vi "whoWins.vi"(2 "white":bool[][](array[boolean]), 3 "black":bool[][](array[boolean])) -> (0 "wWins":bool, 1 "bWins":bool)   [LabVIEW 2014]
panel:
  in  "/wWins":bool
  in  "/bWins":bool
  in  "\\wWins":bool
  in  "\\bWins":bool
  in  "|wWins":bool
  in  "|bWins":bool
  in  "-wWins":bool
  in  "-bWins":bool
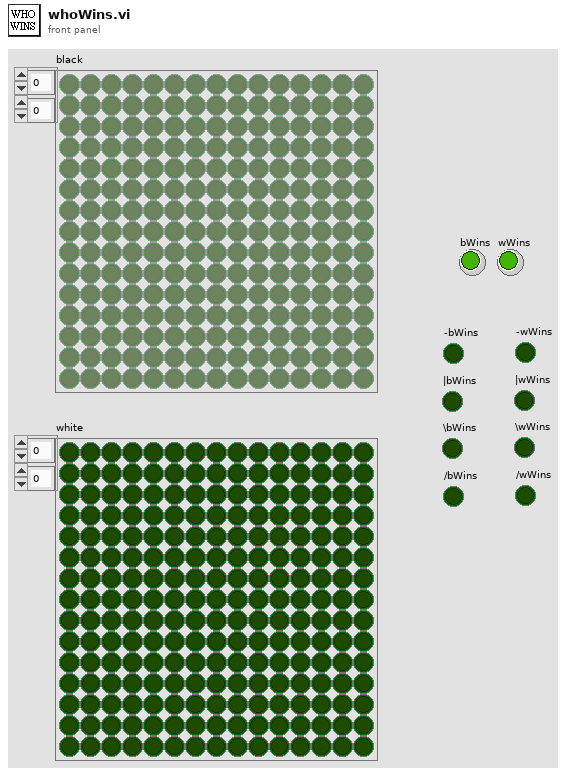
[diagram p1: front panel]
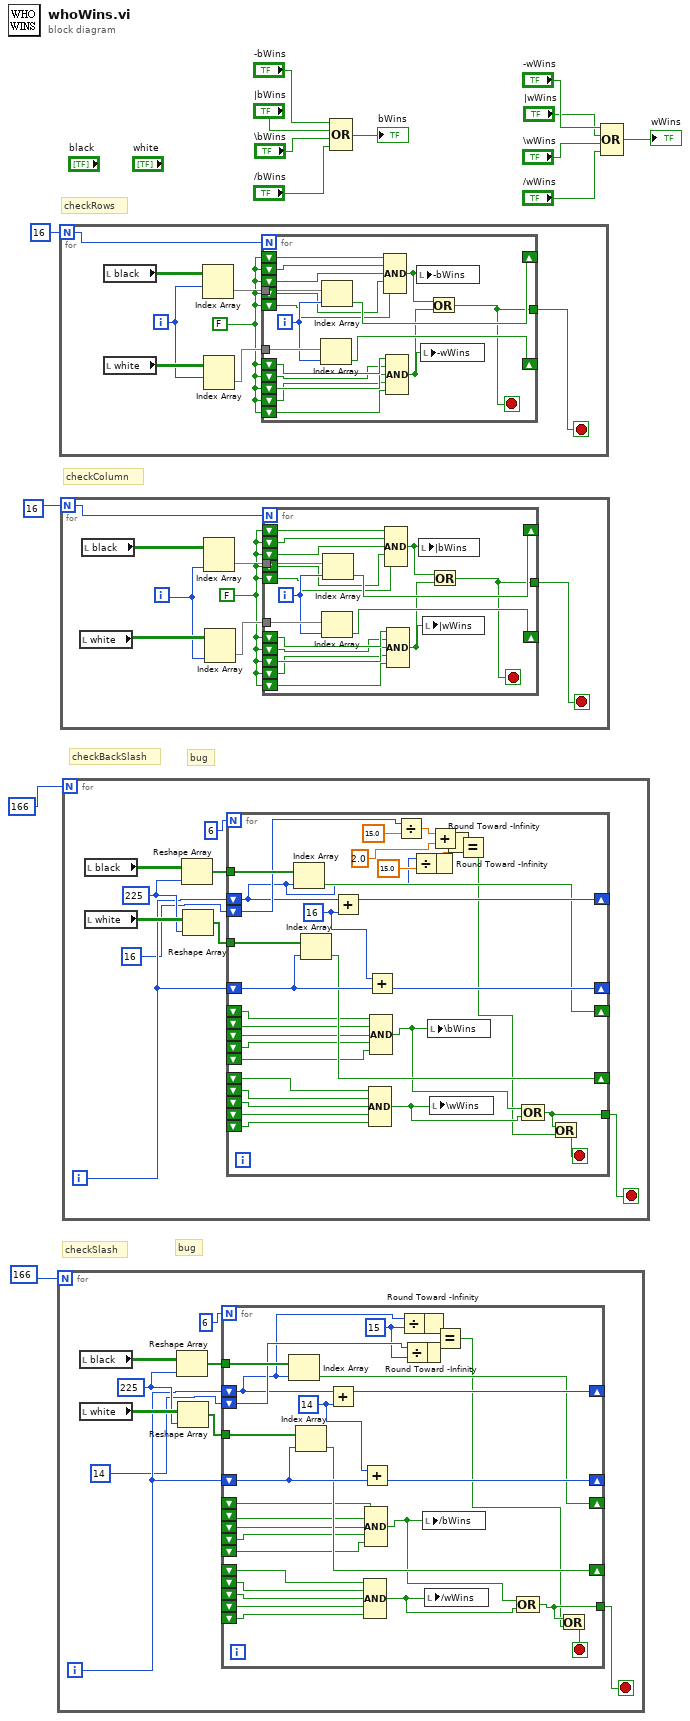
[diagram p0: block diagram]
diagram:
  # "bug"
  # "bug"
  # "checkSlash"
  # "checkBackSlash"
  # "checkColumn"
  # "checkRows"
  n1 = for {
    N: 166 -> [_]
    i -> [w16]
    stop <- w18 stop-if-true
    w21 = 225
    n2 = local read "black"() -> (w23:bool[][])
    n3 = local read "white"() -> (w22:bool[][])
    n4 = Reshape Array(w23, w21) -> (w17:bool[])
    n5 = Reshape Array(w22, w21) -> (w20:bool[])
    n6 = for {
      N: 6 -> [_]
      tunnel: w17 -> [w53]
      tunnel: w20 -> [w52]
      shift-right: [w51] -> _
      shift-left: w16 -> [w29]
      shift-right: [w50] -> _
      shift-left: w16 -> [w48]
      shift-right: [w47] -> _
      shift-left: _ -> [w45]
      shift-right: [w46] -> _
      shift-left: _ -> [w40]
      shift-left: _ -> [w44]
      shift-left: _ -> [w43]
      shift-left: _ -> [w42]
      shift-left: _ -> [w41]
      shift-left: _ -> [w39]
      shift-left: _ -> [w38]
      shift-left: _ -> [w37]
      shift-left: _ -> [w36]
      tunnel: [w33] -> w18
      shift-left: 14 -> [w30]
      stop <- w28 stop-if-true
      w26 = 15
      w49 = 14
      n7 = Index Array(array=w53, index=w29) -> (element=w47:bool)
      n8 = Index Array(array=w52, index=w48) -> (element=w46:bool)
      n9 = Add(x=w29, y=w49) -> (x+y=w51:i32)
      n10 = Add(x=w49, y=w48) -> (x+y=w50:i32)
      n11 = Compound Arithmetic op=AND(w40, w39, w38, w37, w36) -> (w34:bool)
      n12 = Compound Arithmetic op=AND(w45, w44, w43, w42, w41) -> (w35:bool)
      n13 = Divide(x=w29, y=w26) -> (x/y=w32:dbl)
      n14 = Divide(x=w30, y=w26) -> (x/y=w31:dbl)
      n15 = Round Toward -Infinity(1:w31) -> (0:w24:dbl)
      n16 = Round Toward -Infinity(1:w32) -> (0:w25:dbl)
      n17 = local write "/bWins"(w35) -> ()
      n18 = local write "/wWins"(w34) -> ()
      n19 = Equal?(x=w25, y=w24) -> (x = y?=w27:bool)
      n20 = Compound Arithmetic op=OR(w35, w34) -> (w33:bool)
      n21 = Or(x=w33, y=w27) -> (x .or. y?=w28:bool)
    }
  }
  n22 = for {
    N: 16 -> [w55]
    i -> [w59]
    stop <- w56 stop-if-true
    w54 = FALSE
    n23 = local read "black"() -> (w61:bool[][])
    n24 = local read "white"() -> (w60:bool[][])
    n25 = Index Array(array=w61, index (row)=w59) -> (element=w58:bool[])  [unwired: 1 in]
    n26 = Index Array(array=w60, index (row)=w59) -> (element=w57:bool[])  [unwired: 1 in]
    n27 = for {
      N: w55 -> [_]
      tunnel: w58 -> [w78]
      tunnel: w57 -> [w79]
      shift-right: [w76] -> _
      shift-left: w54 -> [w74]
      shift-right: [w75] -> _
      shift-left: w54 -> [w69]
      shift-left: w54 -> [w68]
      shift-left: w54 -> [w67]
      shift-left: w54 -> [w66]
      shift-left: w54 -> [w65]
      shift-left: w54 -> [w73]
      shift-left: w54 -> [w72]
      shift-left: w54 -> [w71]
      shift-left: w54 -> [w70]
      tunnel: [w62] -> w56
      i -> [w77]
      stop <- w62 stop-if-true
      n28 = Index Array(array=w79, index=w77) -> (element=w75:bool)
      n29 = Index Array(array=w78, index=w77) -> (element=w76:bool)
      n30 = Compound Arithmetic op=AND(w74, w73, w72, w71, w70) -> (w64:bool)
      n31 = Compound Arithmetic op=AND(w69, w68, w67, w66, w65) -> (w63:bool)
      n32 = local write "-bWins"(w64) -> ()
      n33 = local write "-wWins"(w63) -> ()
      n34 = Or(x=w64, y=w63) -> (x .or. y?=w62:bool)
    }
  }
  n35 = for {
    N: 16 -> [w81]
    i -> [w82]
    stop <- w85 stop-if-true
    w80 = FALSE
    n36 = local read "white"() -> (w84:bool[][])
    n37 = local read "black"() -> (w83:bool[][])
    n38 = Index Array(array=w83, index (col)=w82) -> (element=w87:bool[])  [unwired: 1 in]
    n39 = Index Array(array=w84, index (col)=w82) -> (element=w86:bool[])  [unwired: 1 in]
    n40 = for {
      N: w81 -> [_]
      tunnel: w87 -> [w104]
      tunnel: w86 -> [w105]
      shift-right: [w102] -> _
      shift-left: w80 -> [w100]
      shift-right: [w101] -> _
      shift-left: w80 -> [w95]
      shift-left: w80 -> [w94]
      shift-left: w80 -> [w93]
      shift-left: w80 -> [w92]
      shift-left: w80 -> [w91]
      shift-left: w80 -> [w99]
      shift-left: w80 -> [w98]
      shift-left: w80 -> [w97]
      shift-left: w80 -> [w96]
      tunnel: [w88] -> w85
      i -> [w103]
      stop <- w88 stop-if-true
      n41 = Index Array(array=w105, index=w103) -> (element=w101:bool)
      n42 = Index Array(array=w104, index=w103) -> (element=w102:bool)
      n43 = Compound Arithmetic op=AND(w100, w99, w98, w97, w96) -> (w90:bool)
      n44 = Compound Arithmetic op=AND(w95, w94, w93, w92, w91) -> (w89:bool)
      n45 = local write "|bWins"(w90) -> ()
      n46 = local write "|wWins"(w89) -> ()
      n47 = Or(x=w90, y=w89) -> (x .or. y?=w88:bool)
    }
  }
  n48 = for {
    N: 166 -> [_]
    i -> [w107]
    stop <- w109 stop-if-true
    w112 = 225
    n49 = local read "black"() -> (w114:bool[][])
    n50 = local read "white"() -> (w113:bool[][])
    n51 = Reshape Array(w114, w112) -> (w108:bool[])
    n52 = Reshape Array(w113, w112) -> (w111:bool[])
    n53 = for {
      N: 6 -> [_]
      tunnel: w108 -> [w147]
      tunnel: w111 -> [w146]
      shift-right: [w145] -> _
      shift-left: w107 -> [w119]
      shift-right: [w144] -> _
      shift-left: w107 -> [w142]
      shift-right: [w141] -> _
      shift-left: _ -> [w139]
      shift-right: [w140] -> _
      shift-left: _ -> [w134]
      shift-left: _ -> [w138]
      shift-left: _ -> [w137]
      shift-left: _ -> [w136]
      shift-left: _ -> [w135]
      shift-left: _ -> [w133]
      shift-left: _ -> [w132]
      shift-left: _ -> [w131]
      shift-left: _ -> [w130]
      tunnel: [w127] -> w109
      shift-left: 16 -> [w120]
      stop <- w118 stop-if-true
      w143 = 16
      n54 = Index Array(array=w147, index=w119) -> (element=w141:bool)
      n55 = Index Array(array=w146, index=w142) -> (element=w140:bool)
      n56 = Add(x=w119, y=w143) -> (x+y=w145:i32)
      n57 = Add(x=w143, y=w142) -> (x+y=w144:i32)
      n58 = Compound Arithmetic op=AND(w134, w133, w132, w131, w130) -> (w128:bool)
      n59 = Compound Arithmetic op=AND(w139, w138, w137, w136, w135) -> (w129:bool)
      n60 = Divide(x=w120, y=15.0) -> (x/y=w122:dbl)
      n61 = Divide(x=w119, y=15.0) -> (x/y=w124:dbl)
      n62 = Round Toward -Infinity(1:w124) -> (0:w115:dbl)
      n63 = local write "\\bWins"(w129) -> ()
      n64 = Add(x=w122, y=2.0) -> (x+y=w123:dbl)
      n65 = local write "\\wWins"(w128) -> ()
      n66 = Round Toward -Infinity(1:w123) -> (0:w116:dbl)
      n67 = Equal?(x=w116, y=w115) -> (x = y?=w117:bool)
      n68 = Compound Arithmetic op=OR(w129, w128) -> (w127:bool)
      n69 = Or(x=w127, y=w117) -> (x .or. y?=w118:bool)
    }
  }
  n70 = Compound Arithmetic op=OR("-bWins", "|bWins", "\\bWins", "/bWins") -> (→"bWins":bool)
  n71 = Compound Arithmetic op=OR("-wWins", "|wWins", "\\wWins", "/wWins") -> (→"wWins":bool)
